vi "Initialize.vi"(6 "Write delay (ms)":u32=1000, 7 "buffer size":i32=4096, 8 "error in (no error)":errorcluster, 10 "Enable? (T)":bool=TRUE, 11 "File path":path) -> (0 "error out":errorcluster, 3 "Logger out":refnum<class "Logger.lvclass">)   [LabVIEW 2013, in "Logger.lvclass"]
doc: "Instantiates a Logger Object which can be used to write data to the location provided by \"File path\" on disk. This method launches a background process which takes care of writing data to disk, allowing an application to call the Log method of the Logger without needing to worry about the effects of a write to disk operation. This is especially important when one wishes to log data from within a time-critical loop.\n\n<b>It is critical that all initialized Logger objects are closed with the Close method.</b> This method signals the background process to stop. If the Close method is not called, the background process will continue to run on the host computer. For this reason, <b>do not abort an application which uses Logger Objects.</b>\n\nNote that <b>the Logger Object is implemented to work by-reference</b>, meaning that copies of an initialized Logger Object will log to the same file internally.\n\nParameters:\n- <file path> \"File path\": specifies location to disk to write the data provided to the Log method.\n- <Boolean> \"Enable? (T)\": specifies whether or not to enable the logger. If False, the background process is not launched, and no logging occurs. Default value is True.\n- <u32> \"Write delay (ms)\": specifies the period between writes to disk by the background process.\n- <i32> \"Buffer size\": specifies the buffer size of the internal queue which passes data provided to the Log method to the background process. A value of \"-1\" indicates an \"infinite\" queue size--see queue documentation for more details.\n\nJared Kirschner, 2012."
uses:
  Logger.lvclass
  Logger.lvclass/Logger.ctl
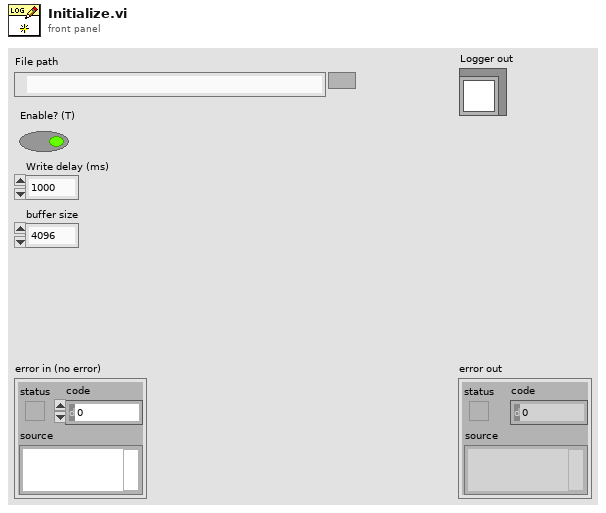
[diagram p1: front panel]
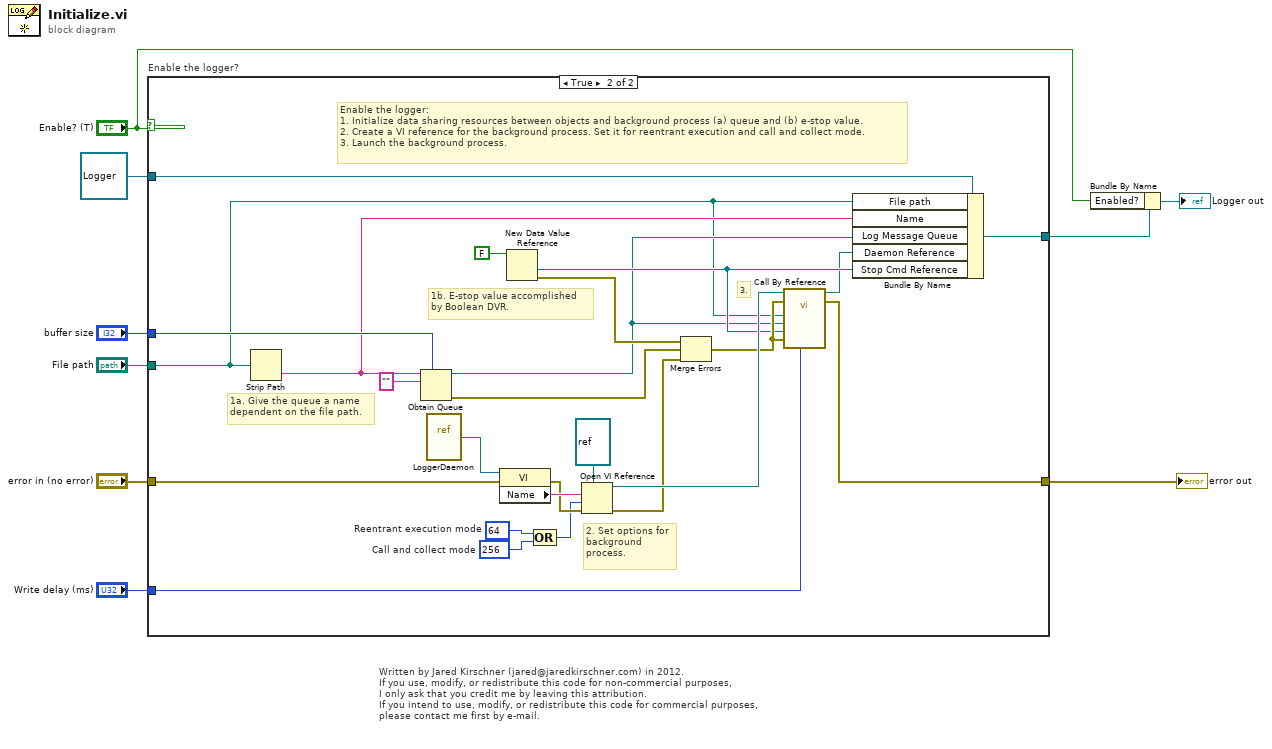
[diagram p0: block diagram]
diagram:
  # "Written by Jared Kirschner (jared@jaredkirschner.com) in 2012.\nIf you use, modify, or redistribute this code for non-commercial purposes,\nI only ask that you credit me by leaving this attribution.\nIf you intend to use, modify, or redistribute this code for commercial purposes,\nplease contact me first by e-mail."
  n1 = case "Enable the logger?" shown="True" "Enable? (T)" {
    tunnel: "buffer size" -> [_ w36]
    tunnel: [w10 w20] -> w8
    tunnel: "error in (no error)" -> [w10 w18]
    tunnel: [w11 w17] -> w3
    tunnel: "Write delay (ms)" -> [_ w16]
    tunnel: "File path" -> [_ w12]
    tunnel: refnum<class "Logger.lvclass"> refnum ("NetworkStreamWriter in") -> [w11 w13]
    frame False {
      # "Do not enable the logger."
    }
    frame True {
      w26 = 64  # Reentrant execution mode
      w27 = 256  # Call and collect mode
      # "3."
      # "2. Set options for\nbackground\nprocess."
      # "1b. E-stop value accomplished\nby Boolean DVR."
      # "Enable the logger:\n1. Initialize data sharing resources between objects and background process (a) queue and (b) e-stop value. \n2. Create a VI reference for the background process. Set it for reentrant execution and call and collect mode.\n3. Launch the background process."
      # "1a. Give the queue a name\ndependent on the file path."
      n2 = Strip Path(path=w12) -> (name=w19:string)  [unwired: 1 out]
      n3 = Obtain Queue(max queue size (-1, unlimited)=w36, name (unnamed)=w19, element data type="" ("name (unnamed)")) -> (queue out=w15:refnum<queue>, error out=w29:errorcluster)  [unwired: 2 in, 1 out]
      n4 = vi-ref "LoggerDaemon.vi"() -> (w35:refnum<vi>)
      n5 = property class="VI"(reference=w35, error in=w18) -> (error out=w31:errorcluster, "Name"=w34:string)  [unwired: 1 out]
      n6 = New Data Value Reference(data value=FALSE) -> (data value reference=w22:refnum<data-value>, error out=w23:errorcluster)  [unwired: 1 in]
      n7 = Compound Arithmetic op=OR(w26, w27) -> (w25:i32)
      n8 = Open VI Reference(type specifier VI Refnum (for type only)=refnum<vi> refnum, vi path=w34, options=w25, error in (no error)=w31) -> (vi reference=w33:refnum<vi>, error out=w30:errorcluster)  [unwired: 2 in]
      n9 = Merge Errors(w23, w29, w30) -> (w28:errorcluster)
      n10 = call-by-ref "?"(reference=w33, error in=w28, "Write delay (ms)"=w16, 8:"error in (no error)"=w28, "Stop Cmd Reference"=w22, "Log Message Queue"=w15, "File path"=w12) -> (reference out=w14:refnum<vi>, error out=w20:errorcluster)  [unwired: 6 in, 1 out]
      n11 = Bundle By Name(cluster=w13, "File path"=w12, "Name"=w19, "Log Message Queue"=w15, "Daemon Reference"=w14, "Stop Cmd Reference"=w22) -> (w17:refnum<class "Logger.lvclass">)
    }
  }
  "error out" <- w8
  n12 = Bundle By Name(cluster=w3, "Enabled?"="Enable? (T)") -> (→"Logger out":refnum<class "Logger.lvclass">)
